vi "ReadPositionVariable.vi"(8 "count":i32, 9 "firstIndex":i32, 10 "HighSpeedEServer":refnum<k24>, 11 "error in (no error)":errorcluster) -> (1 "Axes":i32[][](array[numeric]), 3 "error out":errorcluster)   [LabVIEW 2012, in "UnderAutomation.Yaskawa.lvlib"]
uses:
  UnderAutomation.Yaskawa.lvlib
  C:/Users/fg/Documents/Yaskawa.vi/LabVIEW_2024/UnderAutomation.Yaskawa/lib/UnderAutomation.Yaskawa.dll
  LabVIEW_2024/UnderAutomation.Yaskawa/lib/UnderAutomation.Yaskawa.dll
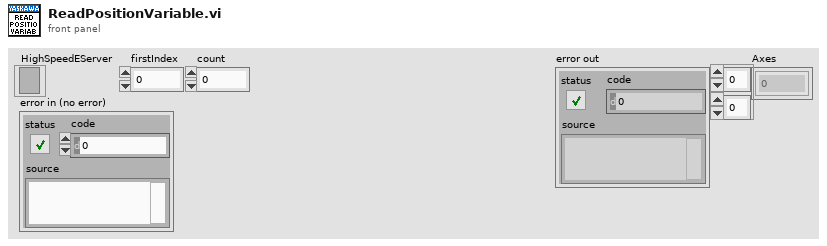
[diagram p1: front panel]
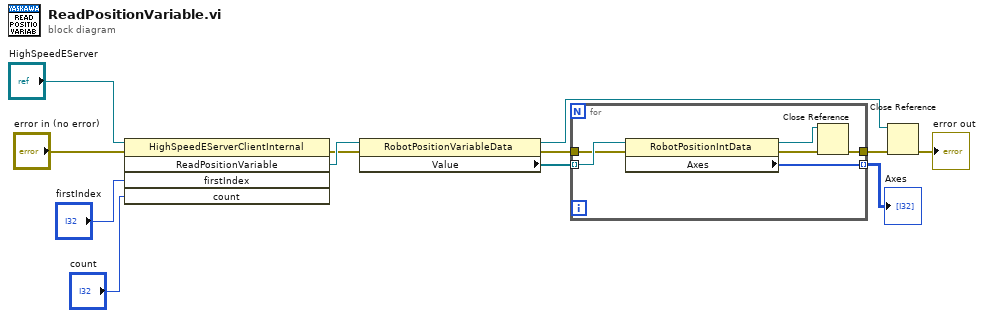
[diagram p0: block diagram]
diagram:
  n1 = invoke class="HighSpeedEServerClientInternal" method="ReadPositionVariable"(reference="HighSpeedEServer", error in="error in (no error)", "firstIndex"="firstIndex", "count"="count") -> (error out=w6:errorcluster, "ReadPositionVariable"=w8:refnum<k24>)  [unwired: 1 in, 3 out]
  n2 = property class="RobotPositionVariableData"(reference=w8, error in=w6) -> (reference out=w7:refnum<k24>, error out=w3:errorcluster, "Value"=w4:refnum<k24>[])
  n3 = for {
    tunnel: w4 -> [w18] mode=indexing
    tunnel: w3 -> [w17]
    tunnel: [w16] -> w2 mode=indexing
    tunnel: [w13] -> w1
    n4 = property class="RobotPositionIntData"(reference=w18, error in=w17) -> (reference out=w15:refnum<k24>, error out=w14:errorcluster, "Axes"=w16:i32[])
    n5 = Close Reference(reference=w15, error in (no error)=w14) -> (error out=w13:errorcluster)
  }
  "Axes" <- w2
  n6 = Close Reference(reference=w7, error in (no error)=w1) -> (error out=→"error out":errorcluster)
